vi "addToActive?.vi"(3 "Baxter in":T2) -> (0 "Active Topics":T1(array[cluster]), 1 "Baxter out":T2)   [LabVIEW 2010]
uses:
  <userlib>/ROSforLV_0.1/ROS/Code/SubVIs/_ROSControl.ctl
  <userlib>/ROSforLV_0.1/ROS/Code/SubVIs/_ROSDirection.ctl
  <userlib>/ROSforLV_0.1/ROS/Code/_ROSDefinition.vi
panel:
  in  "vi reference":refnum<vi>
  in  "error":errorcluster
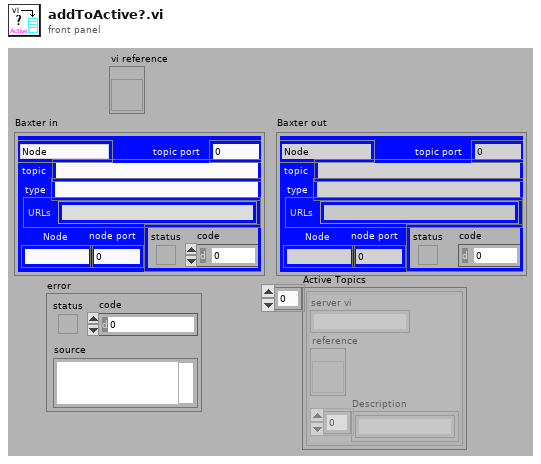
[diagram p1: front panel]
types:
  T1 = cluster{"server vi":string, "reference":refnum<vi>, "Description":string[]}[]
  T2 = typedef "_ROSControl.ctl" = cluster{"topic port":u16, "Node":string, "topic":string, "type":string, "node port":u32, "error ":errorcluster, "Direction":T3, "APIs":string[]}
  T3 = typedef "_ROSDirection.ctl" = enum16{"Node", "Publisher", "Subscriber", "Service Client"}
  T4 = cluster{"vi name":string, "vi reference":refnum<vi>, string[]}
  T5 = cluster{"vi name":string, "vi reference":refnum<vi>, "Description":string[]}[]
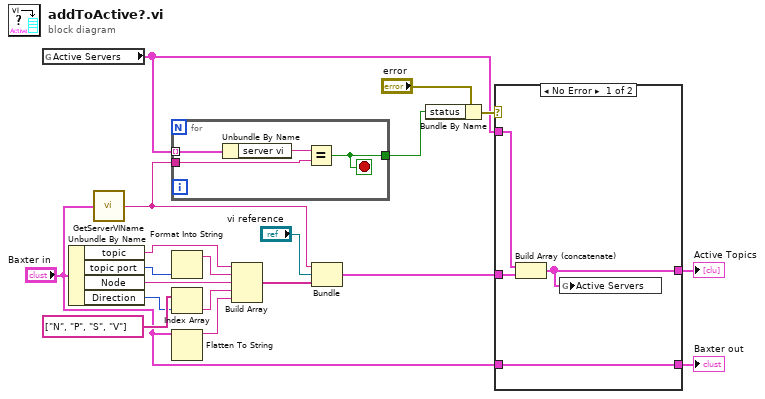
[diagram p0: block diagram]
diagram:
  n1 = global read "_ROSDefinition.vi" "Active Servers"() -> (w1:T1)
  n2 = Unbundle By Name("Baxter in") -> ("topic"=w10:string, "topic port"=w16:u16, "Node"=w11:string, "Direction"=w13:T3)
  n3 = call <userlib>:"GetServerVIName.vi"("Baxter"="Baxter in") -> ("vi name"=w5:string)
  n4 = for {
    tunnel: w1 -> [w23] mode=indexing
    tunnel: w5 -> [w21]
    tunnel: [w20] -> w2
    stop <- w20 stop-if-true
    n5 = Unbundle By Name(w23) -> ("server vi"=w22:string)
    n6 = Equal?(x=w22, y=w21) -> (x = y?=w20:bool)
  }
  n7 = Format Into String(w16) -> (resulting string=w15:string)  [unwired: 3 in, 1 out]
  n8 = Index Array(array=string[] ["N", "P", "S", "V"], index=w13) -> (element=w12:string)
  n9 = Flatten To String(anything="Baxter in") -> (data string=w6:string)  [unwired: 3 in, 2 out]
  n10 = Build Array(w10, w15, w11, w12, w6) -> (w9:string[])
  n11 = Bundle("vi name"=w5, "vi reference"="vi reference", w9) -> (w17:T4)  [unwired: 1 in]
  n12 = Bundle By Name(cluster="error", "status"=w2) -> (w3:errorcluster)
  n13 = case shown="No Error" w3 {
    tunnel: [w26 w29] -> w19
    tunnel: "Baxter in" -> [w26 w29]
    tunnel: w17 -> [w27 _]
    tunnel: [w25 w28] -> w8
    tunnel: w1 -> [w24 w28]
    frame No Error {
      n14 = Build Array (concatenate)(w24, w27) -> (w25:T5)
      n15 = global write "_ROSDefinition.vi" "Active Servers"(w25) -> ()
    }
    frame Error {
    }
  }
  "Baxter out" <- w19
  "Active Topics" <- w8
